vi "fgv_vlp16.vi"(7 "cmd":enum16{"init", "read", "write", "close"}(ring), 8 "error in":errorcluster caption="error out", 11 "send data":string) -> (0 "error out":errorcluster, 3 "receive data":string)   [LabVIEW 2019]
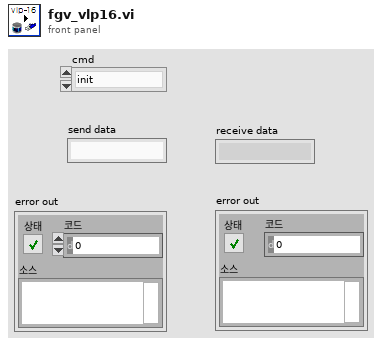
[diagram p1: front panel]
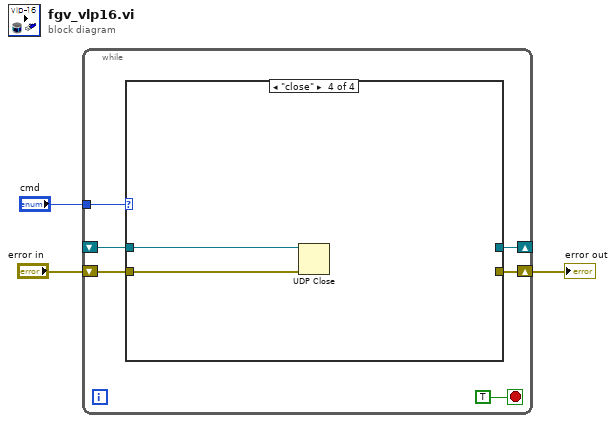
[diagram p0: block diagram]
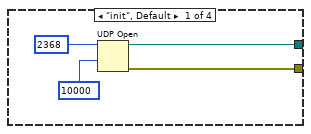
[diagram p2: hidden frame]
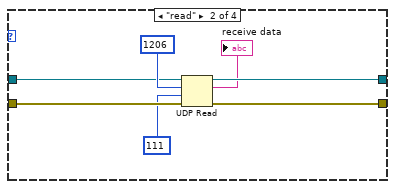
[diagram p3: hidden frame]
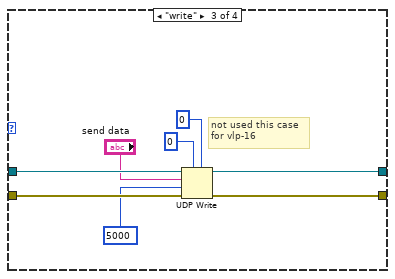
[diagram p4: hidden frame]
diagram:
  n1 = while {
    tunnel: "cmd" -> [w8]
    shift-right: [w6] -> _
    shift-left: _ -> [w4]
    shift-right: [w7] -> w1
    shift-left: "error in" -> [w5]
    stop <- TRUE stop-if-true
    n2 = case shown="\"close\"" w8 {
      tunnel: [w10 w18 w26 _] -> w7
      tunnel: [w11 w19 w25 _] -> w6
      tunnel: w5 -> [_ w17 w27 w29]
      tunnel: w4 -> [_ w16 w28 w30]
      frame "init", Default {
        n3 = UDP Open(9:10000 ("타임아웃 ms (25000)"), 11:u16 2368 ("port")) -> (port=w11:refnum<k16>, 0:w10:errorcluster)  [unwired: 3 in, 1 out]
      }
      frame "read" {
        n4 = UDP Read(connection ID=w16, max size (548)=1206, timeout ms (25000)=111 ("타임아웃 ms (25000)"), 8:w17) -> (data out=→"receive data":string, error out=w18:errorcluster, 3:w19:refnum<k16>)  [unwired: 2 out]
      }
      frame "write" {
        # "not used this case\nfor vlp-16"
        n5 = UDP Write(address=u32 0 ("주소"), port or service name=u16 0 ("포트 또는 서비스 이름"), connection ID=w28, data in="send data", 8:w27, 9:5000 ("타임아웃 ms (25000)")) -> (error out=w26:errorcluster, 3:w25:refnum<k16>)
      }
      frame "close" {
        n6 = UDP Close(connection ID=w30, 8:w29) -> ()  [unwired: 2 out]
      }
    }
  }
  "error out" <- w1
